vi "update.vi"() -> ()   [LabVIEW 2014]
uses:
  <vilib>/Utility/file.llb/Read From Spreadsheet File (DBL).vi
  <vilib>/Utility/file.llb/Write To Spreadsheet File (DBL).vi
  <instrlib>/lake_shore_cryotronics_340/Lake Shore Cryotronics 340/Lake Shore Cryotronics 340.lvlib
  <instrlib>/Agilent 428X Series/Agilent 428X Series.lvlib
panel:
  in  "Auto Level Control (F: Off)":bool
  in  "Manual Output (0.00)":dbl min=0.0 max=100.0 step=0.01 format="%.2f"
  in  "Gain (P) (0.0)":dbl min=0.0 max=1000.0 step=0.1 format="%.1f"
  in  "Heater Range (0: Off)":u16(ring) items=["Off", "1", "2", "3", "4", "5"]
  in  "Loop (0: 1)":u16(ring) items=["1", "2"]
  in  "Reset (I) (0.0)":dbl min=0.0 max=1000.0 step=0.1 format="%.1f"
  in  "Rate (D) (0)":dbl min=0.0 max=1000.0 step=1.0
  in  "Setpoint (0.0)":dbl min=-273.0 max=300000.0 step=0.0001 format="%.4f"
  in  "Delay After Config (1000 ms)":u32=1000 min=1000 max=99999 step=1
  in  "Start Freq (Hz)( 20 Hz)":dbl=20.0 min=20.0 max=30000000.0 step=10.0 format="%^.4e"
  in  "Imp Type (0: CPD)":u32(ring) items=["CPD", "CPQ", "CPG", "CPRP", "CSD", "CSQ", "CSRS", "LPQ", "LPD", "LPG", "LPRP", "LSD", "LSQ", "LSRS", "RX", "ZTD", "ZTR", "GB", "YTD", "YTR"]
  in  "VISA resource name 2":refnum<visa-resource-name>
  out "VISA resource name out":refnum<visa-resource-name>
  out "error out 2":errorcluster
  out "?":cluster{dbl[], dbl[]}[](graph)
  in  "append to file? (new file:F) 2":bool
  in  "append to file? (new file:F) 3":bool
  in  "file path (dialog if empty) 2":path
  in  "file path (dialog if empty) 3":path
  out "Data Status":bool=TRUE
  out "Primary Value":dbl format="%^.4e"
  out "Secondary Value":dbl format="%^.4e"
  in  "file path (dialog if empty) 4":path
  in  "transpose (no:F)":bool
  in  "Input (0: A)":u16(ring) items=["A", "B", "C", "D"]
  out "Celsius Reading":dbl min=-273.16 max=1372.0 step=1e-05 format="%^.5e"
  out "Kelvin Reading":dbl min=0.0 max=1645.0 step=1e-05 format="%^.5e"
  out "Sensor Units Reading":dbl min=-7.5 max=300000.0 step=1e-05 format="%^.5e"
  out "Heater Output":dbl(slide) min=0.0 max=100.0 step=0.01 scale=0.0..100.0 scale format="%.2f"
  out "error out":errorcluster
  in  "append to file? (new file:F)":bool
  in  "file path (dialog if empty)":path
  in  "Configure (F:Don't Config)":bool
  in  "error in (no error)":errorcluster
  in  "VISA resource name":refnum<visa-resource-name>
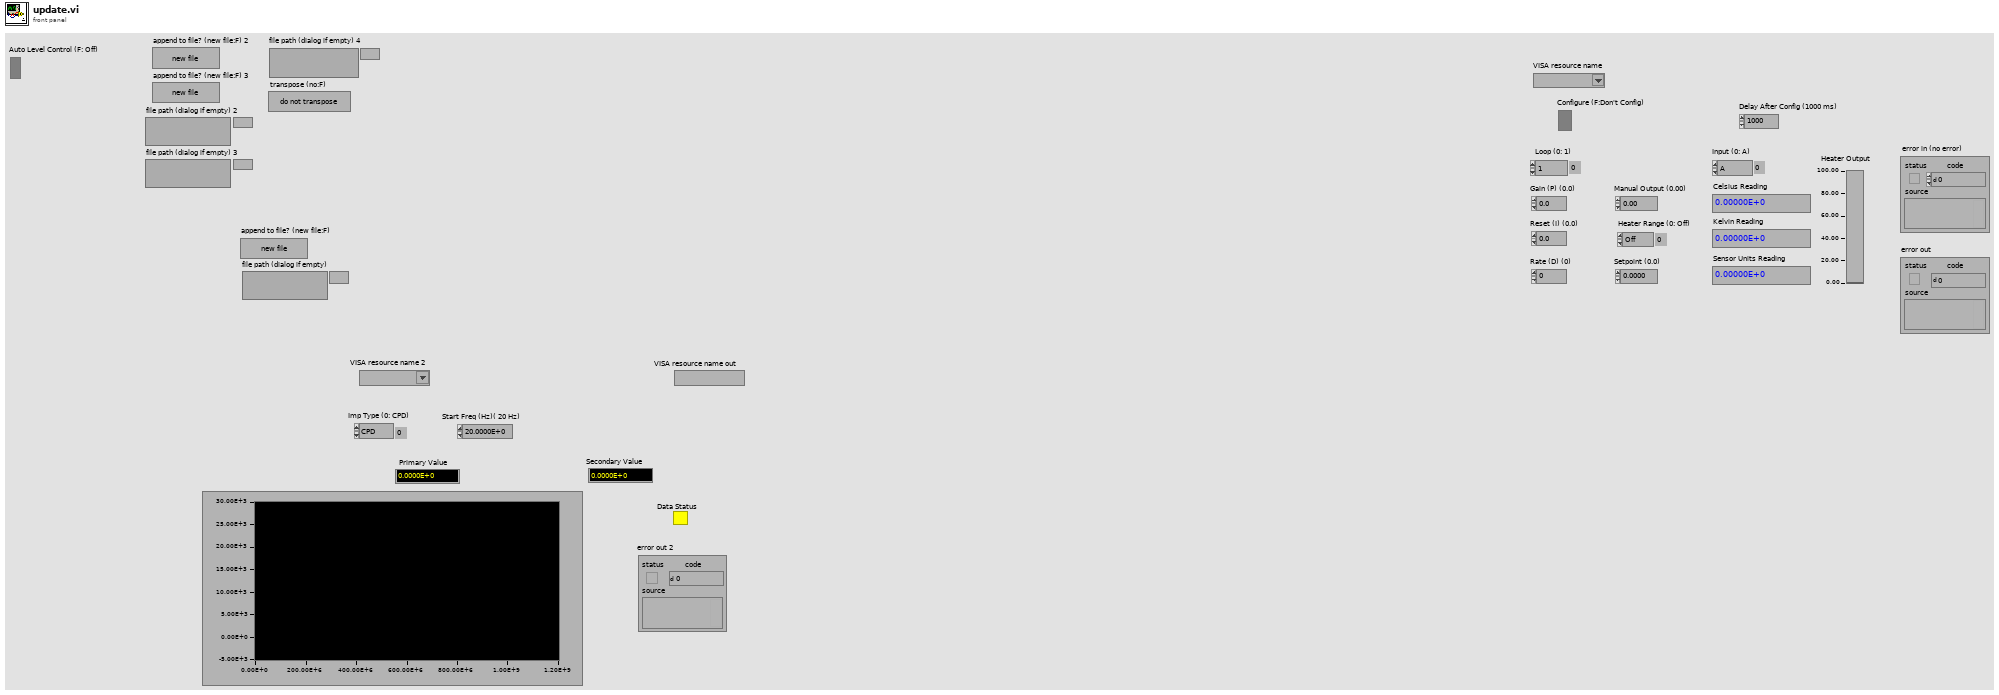
[diagram p1: front panel]
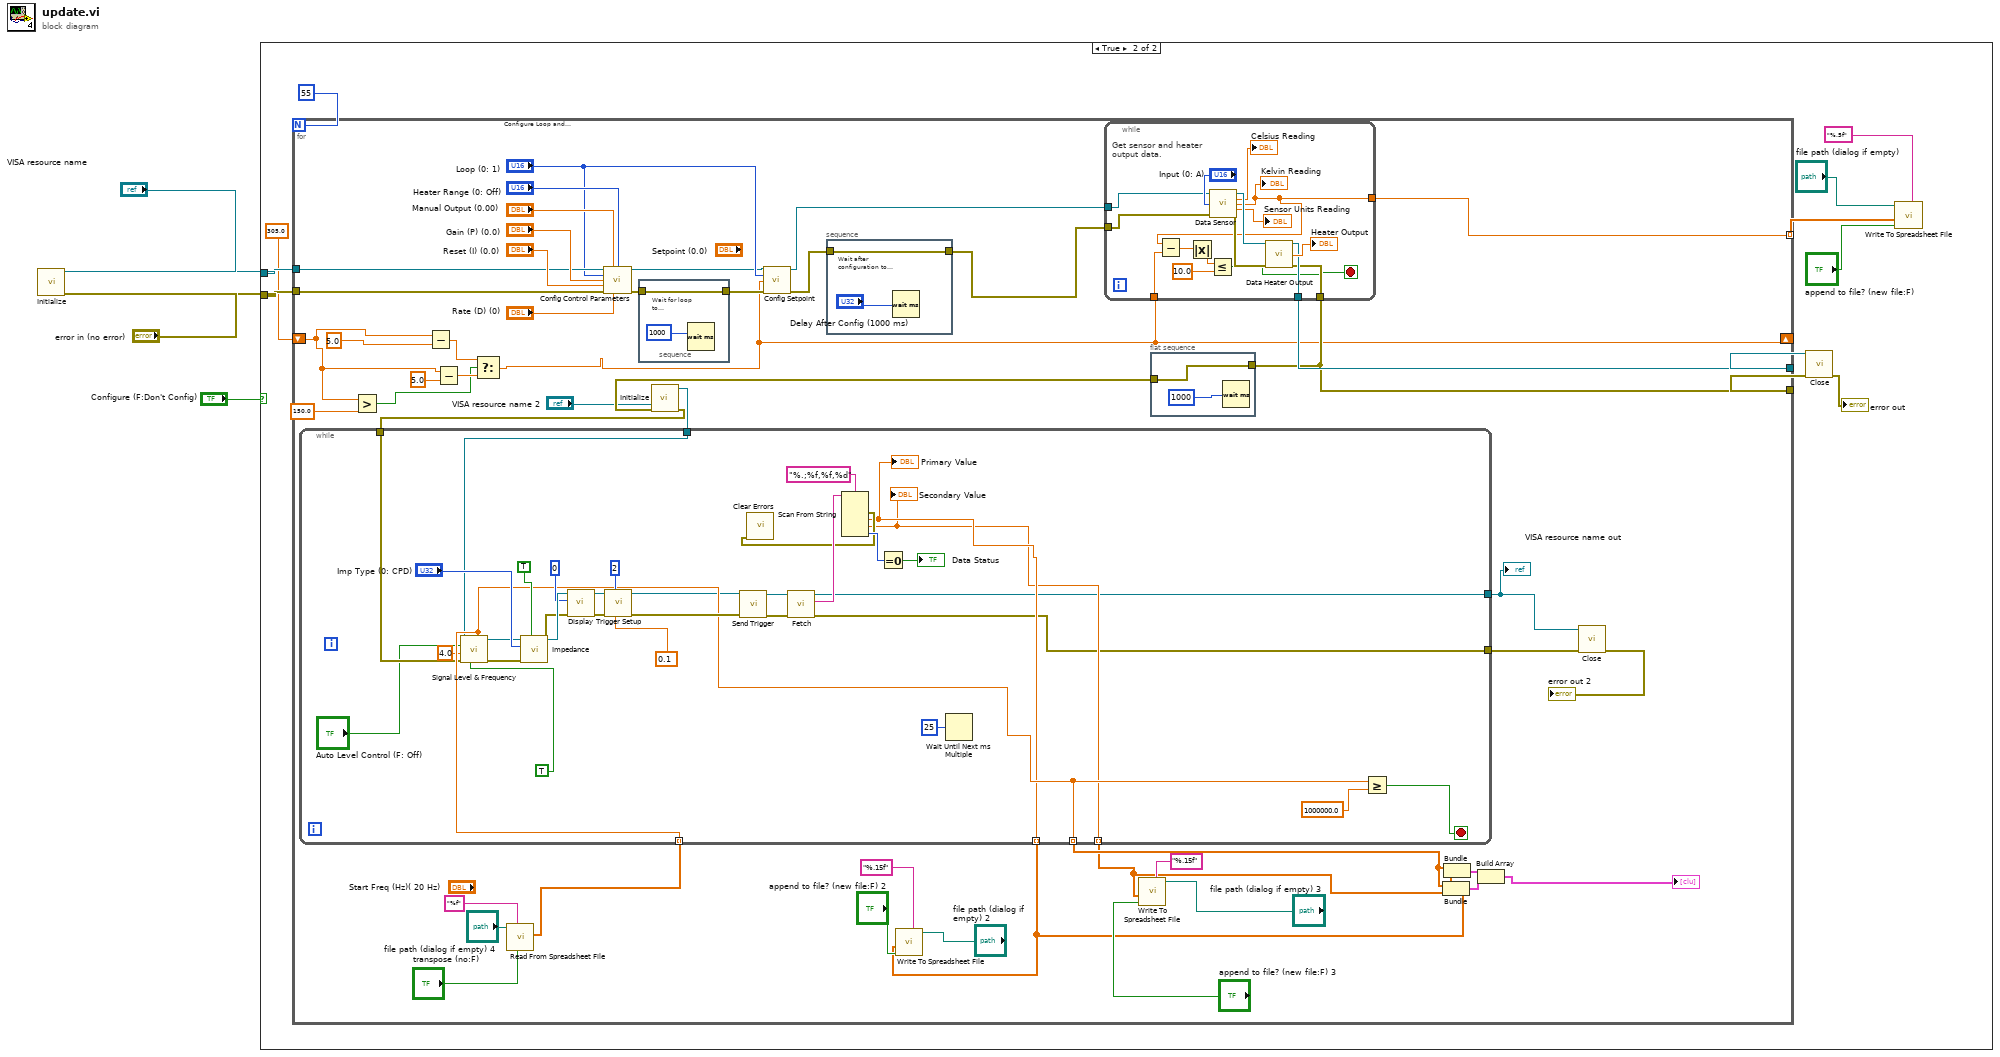
[diagram p0: block diagram]
diagram:
  n1 = call <instrlib>:"Initialize.vi"("VISA resource name"="VISA resource name", "error in (no error)"="error in (no error)") -> ("VISA resource name out"=w1:refnum<visa-resource-name>, "error out"=w2:errorcluster)  [unwired: 12 in]
  n2 = case shown="True" "Configure (F:Don't Config)" {
    tunnel: w2 -> [_ w16]
    tunnel: w1 -> [_ w15]
    frame False {
      # "Do not configure Loop and Setpoint."
    }
    frame True {
      n3 = for {
        N: 55 -> [_]
        shift-right: [w19] -> _
        shift-left: 305.0 -> [w17]
        tunnel: w15 -> [w60]
        tunnel: w16 -> [w64]
        tunnel: [w51] -> w6
        tunnel: [w48] -> w12
        tunnel: [w49] -> w7 mode=indexing
        # "Configure Loop and Setpoint."
        n4 = Greater?(x=w17, y=150.0) -> (0:w20:bool)
        n5 = Subtract(x=w17, y=5.0) -> (x-y=w23:dbl)
        n6 = Subtract(x=w17, y=5.0) -> (x-y=w21:dbl)
        n7 = Select(t=w23, s=w20, f=w21) -> (s? t:f=w19:dbl)
        n8 = call-poly <vilib>:"Read From Spreadsheet File.vi"("transpose (no:F)"="transpose (no:F)", "format (%.3f)"="%f", "file path (dialog if empty)"="file path (dialog if empty) 4") -> ("first row"=w44:dbl[])  [unwired: 4 in, 4 out]
        n9 = call <instrlib>:"Config Control Parameters.vi"("VISA resource name"=w60, "Manual Output (0.00)"="Manual Output (0.00)", "Heater Range (0: Off)"="Heater Range (0: Off)", "Loop (0: 1)"="Loop (0: 1)", "Gain (P) (0.0)"="Gain (P) (0.0)", "Reset (I) (0.0)"="Reset (I) (0.0)", "error in (no error)"=w64, "Rate (D) (0)"="Rate (D) (0)") -> ("VISA resource name out"=w54:refnum<visa-resource-name>, "error out"=w57:errorcluster)  [unwired: 6 in]
        n10 = stacked-sequence {
          tunnel: w57 -> [w118]
          tunnel: [w118] -> w56
          frame #0 {
            # "Wait for loop to \nconfigure."
            n11 = Wait (ms)(milliseconds to wait=u32 1000) -> ()  [unwired: 1 out]
          }
        }
        n12 = call <instrlib>:"Initialize.vi"("error in (no error)"=w28, "VISA resource name"="VISA resource name 2") -> ("error out"=w27:errorcluster, "VISA resource name out"=w25:refnum<visa-resource-name>)  [unwired: 8 in]
        n13 = while {
          tunnel: w44 -> [w77] mode=indexing
          tunnel: [w77] -> w41 mode=indexing
          tunnel: [w76] -> w32 mode=indexing
          tunnel: [w75] -> w33 mode=indexing
          tunnel: [w72] -> w31
          tunnel: [w71] -> w30
          tunnel: w27 -> [w70]
          tunnel: w25 -> [w69]
          stop <- w88 stop-if-true
          n14 = call <instrlib>:"Signal Level & Frequency.vi"("Frequency Value (Hz) (100KHz)"=w77, "Oscillator Select (T: Voltage)"=TRUE, "error in (no error)"=w70, "Voltage Level (V) (5mV)"=4.0, "Auto Level Control (F: Off)"="Auto Level Control (F: Off)", "VISA resource name"=w69) -> ("error out"=w79:errorcluster, "VISA resource name out"=w74:refnum<visa-resource-name>)  [unwired: 4 in]
          n15 = call <instrlib>:"Impedance.vi"("Auto Range (F: Off)"=TRUE ("Auto Range (Off:F)"), "error in (no error)"=w79, "Imp Type (0: CPD)"="Imp Type (0: CPD)", "VISA resource name"=w74) -> ("error out"=w94:errorcluster, "VISA resource name out"=w97:refnum<visa-resource-name>)  [unwired: 6 in]
          n16 = call <instrlib>:"Display.vi"("error in (no error)"=w94, "Display Page (0: Measurement)"=u32 0 ("Display Page (Measurment:0)"), "VISA resource name"=w97) -> ("error out"=w95:errorcluster, "VISA resource name out"=w96:refnum<visa-resource-name>)  [unwired: 7 in]
          n17 = call <instrlib>:"Trigger Setup.vi"("Delay Value (s) (0.0)"=0.1, "Trigger Source (0: Internal)"=u32 2 ("Trigger Source (Internal:0)"), "error in (no error)"=w95, "VISA resource name"=w96) -> ("error out"=w78:errorcluster, "VISA resource name out"=w73:refnum<visa-resource-name>)  [unwired: 6 in]
          n18 = call <instrlib>:"Send Trigger.vi"("error in (no error)"=w78, "VISA resource name"=w73) -> ("error out"=w68:errorcluster, "VISA resource name out"=w82:refnum<visa-resource-name>)  [unwired: 8 in]
          n19 = call <instrlib>:"Fetch.vi"("error in (no error)"=w68, "VISA resource name"=w82) -> ("error out"=w71:errorcluster, "Returned Data"=w83:string, "VISA resource name out"=w72:refnum<visa-resource-name>)  [unwired: 7 in]
          n20 = Scan From String(format string="%.;%f,%f,%d", input string=w83) -> (error out=w80:errorcluster, output 1=w76:dbl, output 2=w75:dbl, output 3=w85:i32)  [unwired: 5 in, 2 out]
          "Primary Value" <- w76
          "Secondary Value" <- w75
          n21 = call <vilib>:"Clear Errors.vi"("error in (no error)"=w80) -> ()  [unwired: 5 in, 2 out]
          n22 = Equal To 0?(x=w85) -> (x = 0?=→"Data Status":bool)
          n23 = Wait Until Next ms Multiple(millisecond multiple=u32 25) -> ()  [unwired: 1 out]
          n24 = Greater Or Equal?(x=w77, y=1000000.0) -> (x >= y?=w88:bool)
        }
        "VISA resource name out" <- w31
        n25 = call <instrlib>:"Config Setpoint.vi"("VISA resource name"=w54, "Loop (0: 1)"="Loop (0: 1)", "Setpoint (0.0)"=w19, "error in (no error)"=w56) -> ("VISA resource name out"=w52:refnum<visa-resource-name>, "error out"=w53:errorcluster)  [unwired: 10 in]
        n26 = stacked-sequence {
          tunnel: w53 -> [w117]
          tunnel: [w117] -> w50
          frame #0 {
            # "Wait after configuration to\nread data."
            n27 = Wait (ms)(milliseconds to wait="Delay After Config (1000 ms)") -> ()  [unwired: 1 out]
          }
        }
        n28 = call-poly <vilib>:"Write To Spreadsheet File.vi"("format (%.3f)"="%.15f", "append to file? (new file:F)"="append to file? (new file:F) 2", "1D data"=w32, "file path (dialog if empty)"="file path (dialog if empty) 2") -> ()  [unwired: 4 in, 1 out]
        n29 = while {
          tunnel: [w105] -> w49
          tunnel: w52 -> [w109]
          tunnel: [w108] -> w51
          tunnel: [w107] -> w48
          tunnel: w50 -> [w106]
          tunnel: w19 -> [w104]
          stop <- w100 stop-if-true
          # "Get sensor and heater\noutput data."
          n30 = call <instrlib>:"Data Sensor.vi"("VISA resource name"=w109, "Input (0: A)"="Input (0: A)", "error in (no error)"=w106) -> ("VISA resource name out"=w115:refnum<visa-resource-name>, "Celsius Reading"=→"Celsius Reading":dbl, "Kelvin Reading"=w105:dbl, "Sensor Units Reading"=→"Sensor Units Reading":dbl, "error out"=w111:errorcluster)  [unwired: 8 in]
          "Kelvin Reading" <- w105
          n31 = Subtract(x=w105, y=w104) -> (x-y=w103:dbl)
          n32 = Absolute Value(x=w103) -> (abs(x)=w102:dbl)
          n33 = Less Or Equal?(x=w102, y=10.0) -> (x <= y?=w100:bool)
          n34 = call <instrlib>:"Data Heater Output.vi"("VISA resource name"=w115, "error in (no error)"=w111) -> ("VISA resource name out"=w108:refnum<visa-resource-name>, "Heater Output"=→"Heater Output":dbl, "error out"=w107:errorcluster)  [unwired: 11 in]
        }
        n35 = call-poly <vilib>:"Write To Spreadsheet File.vi"("format (%.3f)"="%.15f", "append to file? (new file:F)"="append to file? (new file:F) 3", "1D data"=w33, "file path (dialog if empty)"="file path (dialog if empty) 3") -> ()  [unwired: 4 in, 1 out]
        n36 = flat-sequence {
          tunnel: w48 -> [w99]
          tunnel: [w99] -> w28
          frame #0 {
            n37 = Wait (ms)(milliseconds to wait=u32 1000) -> ()  [unwired: 1 out]
          }
        }
        n38 = Bundle(w41, w33) -> (w42:cluster{dbl[], dbl[]})  [unwired: 1 in]
        n39 = Bundle(w41, w32) -> (w43:cluster{dbl[], dbl[]})  [unwired: 1 in]
        n40 = Build Array(w43, w42) -> (→"?":cluster{dbl[], dbl[]}[])
        n41 = call <instrlib>:"Close.vi"("error in (no error)"=w30, "VISA resource name"=w31) -> ("error out"=→"error out 2":errorcluster)  [unwired: 9 in]
      }
      n42 = call <instrlib>:"Close.vi"("VISA resource name"=w6, "error in (no error)"=w12) -> ("error out"=→"error out":errorcluster)  [unwired: 13 in]
      n43 = call-poly <vilib>:"Write To Spreadsheet File.vi"("format (%.3f)"="%.5f", "append to file? (new file:F)"="append to file? (new file:F)", "1D data"=w7, "file path (dialog if empty)"="file path (dialog if empty)") -> ()  [unwired: 4 in, 1 out]
    }
  }
